vi "crop_rectangular.vi"(10 "dbl_ar_crop_correction":dbl[](array[numeric])=[0.0, 0.0, 0.0, 0.0], 11 "image_in":T1) -> (2 "crop boundaries":dbl[](array[numeric]), 3 "cropped image out":T1)   [LabVIEW 2011]
uses:
  <vilib>/vision/Image Controls.llb/IMAQ Image.ctl
  <vilib>/vision/NI_Vision_Development_Module.lvlib
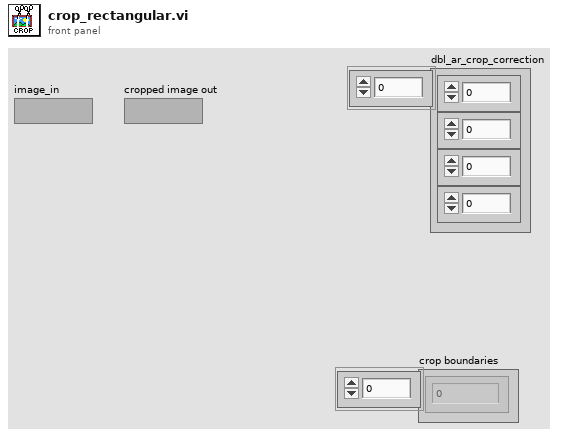
[diagram p1: front panel]
types:
  T1 = typedef "IMAQ Image.ctl" = refnum<image>
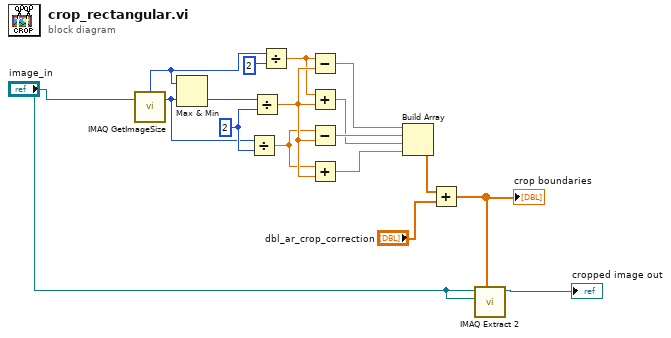
[diagram p0: block diagram]
diagram:
  w15 = 2 ("y")
  n1 = call "IMAQ GetImageSize"("Image"="image_in") -> ("Y Resolution"=w7:i32, "X Resolution"=w5:i32)  [unwired: 3 in, 1 out]
  n2 = Max & Min(x=w5, y=w7) -> (min(x,y)=w14:i32)  [unwired: 1 out]
  n3 = Divide(x=w7, y=w15) -> (x/y=w9:dbl)
  n4 = Divide(x=w14, y=w15) -> (x/y=w13:dbl)
  n5 = Divide(x=w5, y=2) -> (x/y=w8:dbl)
  n6 = Subtract(x=w8, y=w13) -> (x-y=w10:dbl)
  n7 = Add(x=w8, y=w13) -> (x+y=w11:dbl)
  n8 = Subtract(x=w9, y=w13) -> (x-y=w17:dbl)
  n9 = Add(x=w9, y=w13) -> (x+y=w16:dbl)
  n10 = Build Array(w10, w17, w11, w16) -> (w3:dbl[])
  n11 = Add(x=w3, y="dbl_ar_crop_correction") -> (x+y=w4:dbl[])
  "crop boundaries" <- w4
  n12 = call "IMAQ Extract 2"("Optional Rectangle"=w4, "Image Dst"="image_in", "Image Src"="image_in") -> ("Image Dst Out"=→"cropped image out":T1)  [unwired: 7 in, 1 out]
